vi "Change ILC Booster Valve Gain.vi"(0 "Model in":refnum<class "Model.lvclass">, 11 "error in (no error)":errorcluster) -> (4 "Model out":refnum<class "Model.lvclass">, 15 "error out":errorcluster)   [LabVIEW 2016, in "Model.lvclass"]
uses:
  Model.lvclass
  Model.lvclass/Model.ctl
  Common_RT_FAILC/FAILC/FAILC.lvclass/FAILC.ctl
  Common_RT_Modbus/DynamicFrameParser/DynamicFrameParser.lvclass
  Modbus/DesktopModbus/DesktopModbus.lvclass
  Common_RT_FAILC/FAILC/FAILC.lvclass
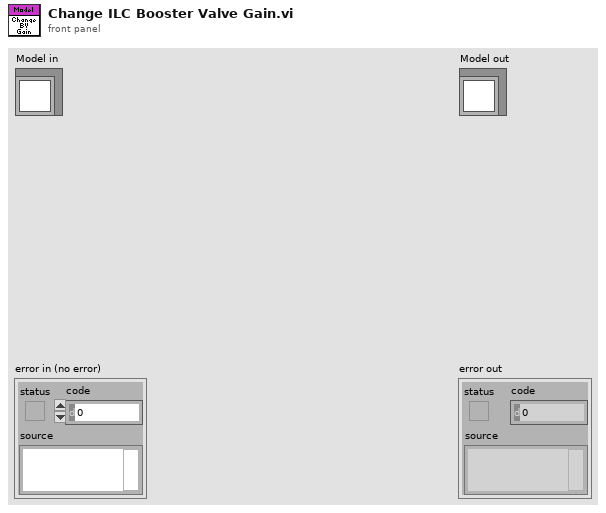
[diagram p1: front panel]
types:
  T1 = typedef "RTFAILC.lvlib/FAData.ctl" = cluster{"Constants":T2, "Command":T3, "Telemetry":T4, "Responses":T5, "Timings":T7}
  T2 = typedef "RTFAILC.lvlib/FAConstants.ctl" = cluster{"ID":i16}
  T3 = typedef "RTFAILC.lvlib/FACommand.ctl" = cluster{"AxialSetPoint":i32, "LateralSetPoint":i32, "AxialBoosterValveGain":sgl, "LateralBoosterValveGain":sgl}
  T4 = typedef "RTFAILC.lvlib/FATelemetry.ctl" = cluster{"ILCFault":bool, "BroadcastCounter":u8, "AxialLoadCellForce":sgl, "LateralLoadCellForce":sgl, "AxialBoosterValveGain":sgl, "LateralBoosterValveGain":sgl}
  T5 = typedef "RTFAILC.lvlib/FAResponses.ctl" = cluster{"BoosterValveGain":T6, "ReadBoosterValveGain":T6, "SetForce":T6, "ForceAndStatus":T6}
  T6 = typedef "RTModbus.lvlib/ExceptionCodes.ctl" = u16
  T7 = typedef "RTFAILC.lvlib/FATimings.ctl" = cluster{"BroadcastSetForce":u32, "BoosterValveGain":u32, "FreezeSensorValues":u32, "ForceAndStatus":u32, "ReadBoosterValveGain":u32, "SetForce":u32}
  T8 = typedef "RTModbus.lvlib/TxFrame.ctl" = cluster{"Data":u8[], "WaitForTrigger":bool, "WaitForRx":u16, "TriggerIRQ":bool, "DelayMicroseconds":u16, "DelayMilliseconds":u16, "Timestamp":bool}
  T9 = typedef "RTModbus.lvlib/RxFrame.ctl" = cluster{"Data":u8[], "Timestamp":u64}
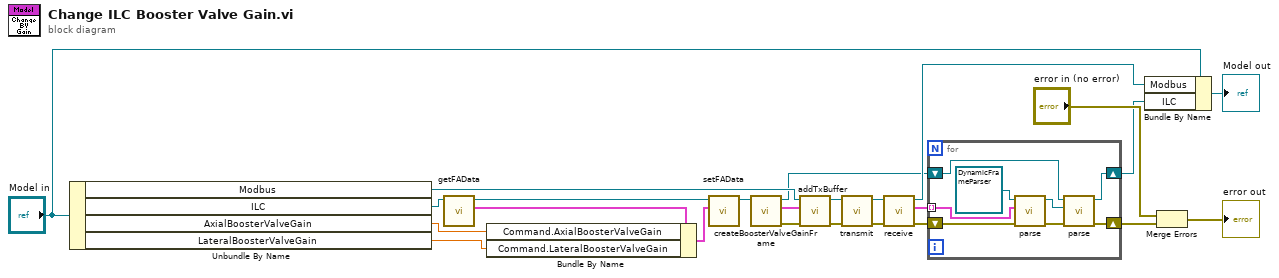
[diagram p0: block diagram]
diagram:
  n1 = Unbundle By Name("Model in") -> ("Modbus"=w23:refnum<class "DesktopModbus.lvclass">, "ILC"=w10:refnum<class "FAILC.lvclass">, "AxialBoosterValveGain"=w8:sgl, "LateralBoosterValveGain"=w7:sgl)
  n2 = call "getFAData.vi"("FAILC in"=w10) -> ("FAData"=w9:T1, "FAILC out"=w5:refnum<class "FAILC.lvclass">)  [unwired: 9 in]
  n3 = Bundle By Name(cluster=w9, "Command.AxialBoosterValveGain"=w8, "Command.LateralBoosterValveGain"=w7) -> (w6:T1)
  n4 = call "setFAData.vi"("FAData"=w6, "FAILC in"=w5) -> ("FAILC out"=w4:refnum<class "FAILC.lvclass">)  [unwired: 9 in]
  n5 = call "createBoosterValveGainFrame.vi"("FAILC in"=w4) -> ("error out"=w1:errorcluster, "TxFrame"=w2:T8, "FAILC out"=w3:refnum<class "FAILC.lvclass">)  [unwired: 8 in]
  n6 = call-dynamic "addTxBuffer.vi"("error in (no error)"=w1, "TxFrame"=w2, "DesktopModbus in"=w23) -> ("error out"=w20:errorcluster, "DesktopModbus out"=w22:refnum<class "DesktopModbus.lvclass">)  [unwired: 7 in]
  n7 = call-dynamic "transmit.vi"("error in (no error)"=w20, "DesktopModbus in"=w22) -> ("error out"=w19:errorcluster, "DesktopModbus out"=w21:refnum<class "DesktopModbus.lvclass">)  [unwired: 8 in]
  n8 = call-dynamic "receive.vi"("error in (no error)"=w19, "DesktopModbus in"=w21) -> ("error out"=w13:errorcluster, "Data"=w14:T9[], "DesktopModbus out"=w16:refnum<class "DesktopModbus.lvclass">)  [unwired: 7 in]
  n9 = for {
    tunnel: w14 -> [w30] mode=indexing
    shift-right: [w27] -> w12
    shift-left: w13 -> [w29]
    shift-right: [w25] -> w11
    shift-left: w3 -> [w26]
    n10 = call "parse.vi"("error in (no error)"=w29, "RxFrame"=w30, "FrameParser in"=refnum<class "DynamicFrameParser.lvclass"> refnum ("RTModbus.lvlib:DynamicFrameParser.lvclass")) -> ("error out"=w28:errorcluster, "FrameParser out"=w32:refnum<class "DynamicFrameParser.lvclass">)  [unwired: 7 in]
    n11 = call-dynamic "parse.vi"("error in (no error)"=w28, "DynamicFrameParser"=w32, "FAILC in"=w26) -> ("error out"=w27:errorcluster, "FAILC out"=w25:refnum<class "FAILC.lvclass">)  [unwired: 6 in, 1 out]
  }
  n12 = Bundle By Name(cluster="Model in", "Modbus"=w16, "ILC"=w11) -> (→"Model out":refnum<class "Model.lvclass">)
  n13 = Merge Errors("error in (no error)", w12) -> (→"error out":errorcluster)
